vi "Main.vi"() -> ()   [LabVIEW 2014]
uses:
  <vilib>/regexp/Match Regular Expression.xnode
panel:
  out "Disticts":dbl
  in  "Find # Distincts":bool
  out "Symbol":string
  in  "Find Symbol":bool
  in  "Clear":bool
  in  "Stop Button":bool
  in  "Validate":bool
  out "Valid?":bool
  in  "Element symbol":string
  in  "Element Name":string
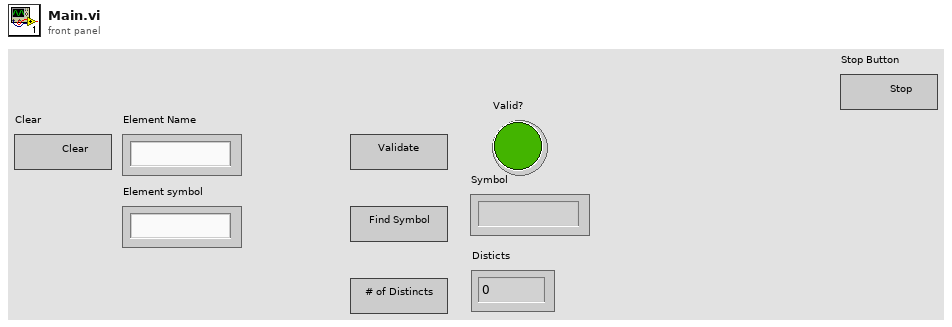
[diagram p1: front panel]
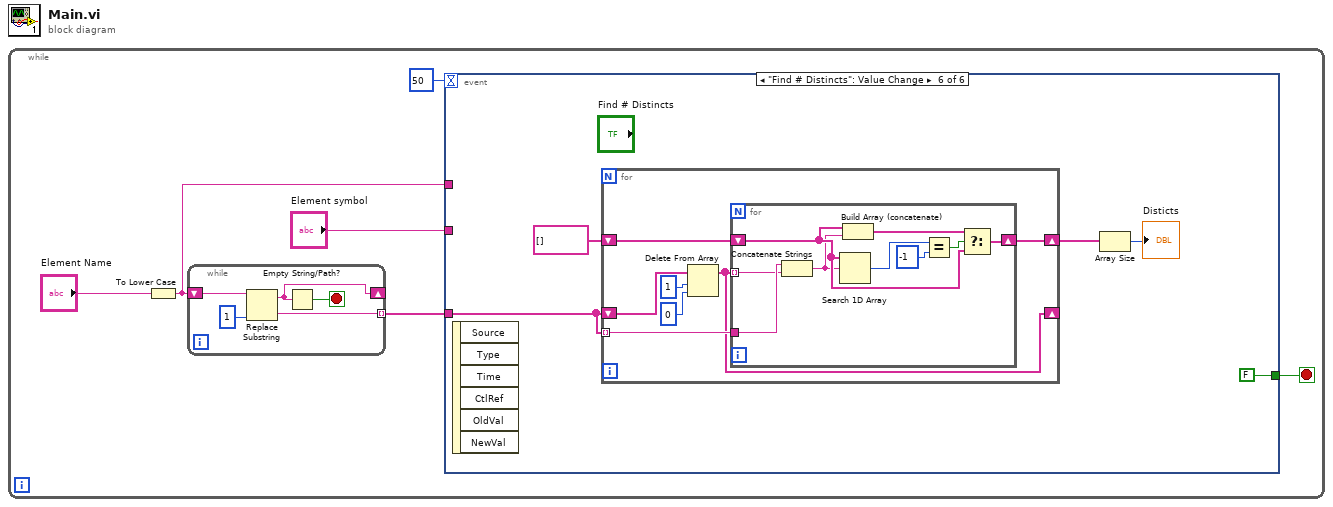
[diagram p0: block diagram]
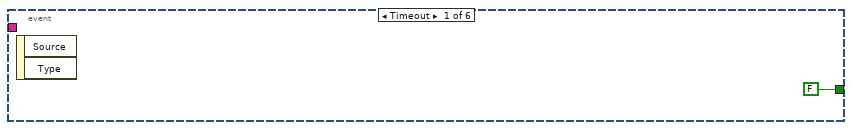
[diagram p2: hidden frame]
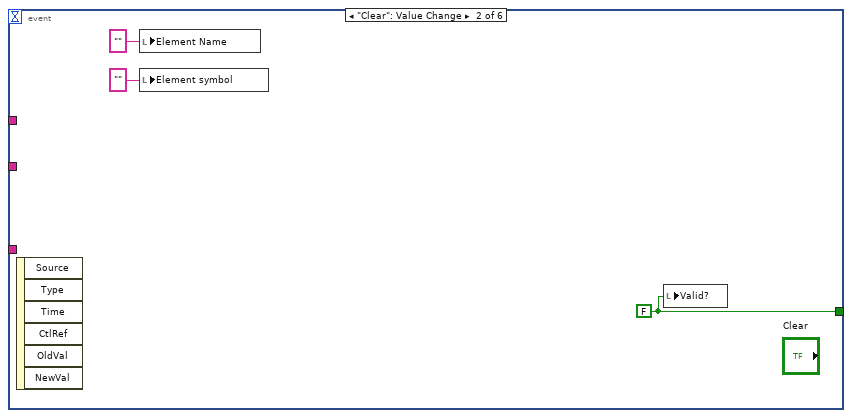
[diagram p3: hidden frame]
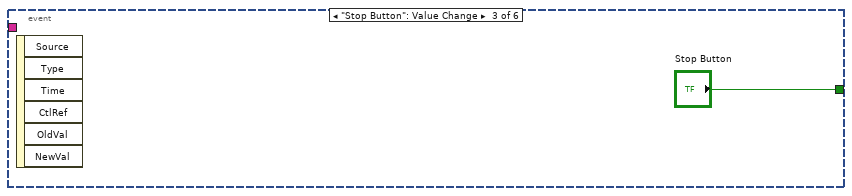
[diagram p4: hidden frame]
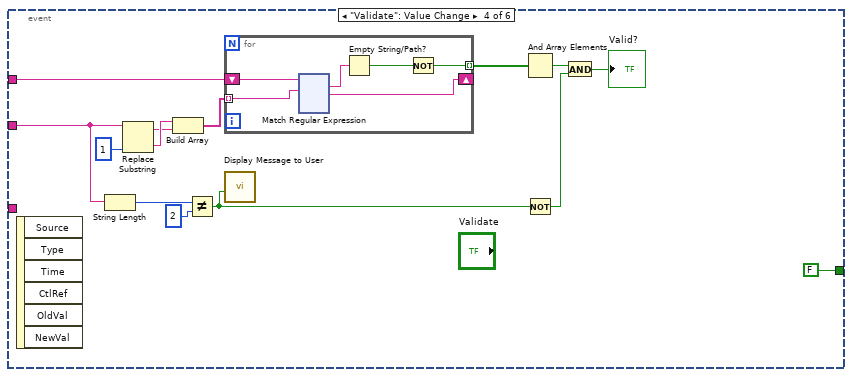
[diagram p5: hidden frame]
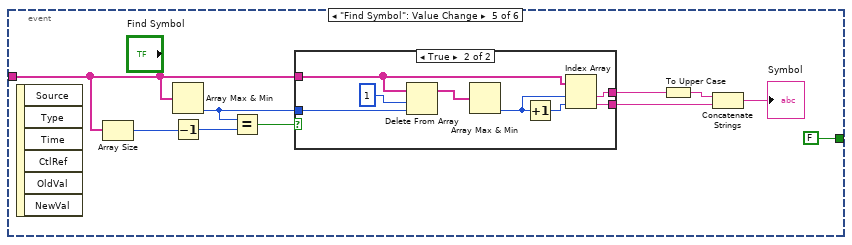
[diagram p6: hidden frame]
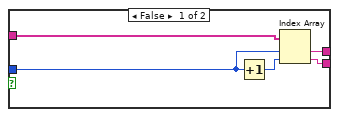
[diagram p7: hidden frame]
diagram:
  n1 = while {
    stop <- w6 stop-if-true
    n2 = To Lower Case(string="Element Name") -> (all lower case string=w2:string)
    n3 = while {
      shift-right: [w8] -> _
      shift-left: w2 -> [w11]
      tunnel: [w9] -> w1 mode=indexing
      stop <- w7 stop-if-true
      n4 = Replace Substring(2:1 ("length (len. of substring)"), 5:w11) -> (0:w9:string, 1:w8:string)  [unwired: 2 in]
      n5 = Empty String/Path?(string/path=w8) -> (empty?=w7:bool)
    }
    n6 = event shown="[5] \"Find # Distincts\": Value Change" {
      selector: _ -> [_ _ _ _ _ _]
      dyn-events: _ -> [_ _ _ _ _ _]
      timeout: 50 -> [_ _ _ _ _ _]
      tunnel: [FALSE w15 "Stop Button" FALSE ("Stop Button") FALSE ("Stop Button") FALSE ("Stop Button")] -> w6
      tunnel: w2 -> [_ _ _ w18 _ _]
      tunnel: "Element symbol" -> [_ _ _ w17 _ _]
      tunnel: w1 -> [_ _ _ _ w151 w177]
      event Timeout {
        n7 = event-data() -> ()  [unwired: 1 in, 2 out]
      }
      event "Clear": Value Change {
        w15 = FALSE
        n8 = event-data() -> ()  [unwired: 1 in, 6 out]
        n9 = local write "Element Name"("" ("Element Name")) -> ()
        n10 = local write "Element symbol"("" ("Element symbol")) -> ()
        n11 = local write "Valid?"(w15) -> ()
      }
      event "Stop Button": Value Change {
        n12 = event-data() -> ()  [unwired: 1 in, 6 out]
      }
      event "Validate": Value Change {
        n13 = event-data() -> ()  [unwired: 1 in, 6 out]
        n14 = String Length(string=w17) -> (length=w24:i32)
        n15 = Replace Substring(2:1 ("length (len. of substring)"), 5:w17) -> (0:w29:string, 1:w28:string)  [unwired: 2 in]
        n16 = Build Array(w29, w28) -> (w27:string[])
        n17 = Not Equal?(x=w24, y=2) -> (x != y?=w22:bool)
        n18 = for {
          tunnel: w27 -> [w34] mode=indexing
          shift-right: [w35] -> _
          shift-left: w18 -> [w36]
          tunnel: [w31] -> w26 mode=indexing
          n19 = xnode "Match Regular Expression"("input string"=w36, "regular expression"=w34) -> ("whole match"=w33:string, "after match"=w35:string)  [unwired: 4 in, 3 out]
          n20 = Empty String/Path?(string/path=w33) -> (empty?=w32:bool)
          n21 = Not(x=w32) -> (.not. x?=w31:bool)
        }
        n22 = call "Display Message to User"("Enable"=w22) -> ()  [unwired: 9 in, 2 out]
        n23 = And Array Elements(Boolean array=w26) -> (logical AND=w21:bool)
        n24 = Not(x=w22) -> (.not. x?=w20:bool)
        n25 = And(x=w21, y=w20) -> (x .and. y?=→"Valid?":bool)
      }
      event "Find Symbol": Value Change {
        n26 = event-data() -> ()  [unwired: 1 in, 6 out]
        n27 = Array Size(array=w151) -> (size(s)=w159:i32)
        n28 = Array Max & Min(array=w151) -> (min index (indices)=w157:i32)  [unwired: 3 out]
        n29 = Decrement(x=w159) -> (x-1=w158:i32)
        n30 = Equal?(x=w157, y=w158) -> (x = y?=w156:bool)
        n31 = case shown="True" w156 {
          tunnel: w151 -> [w161 w170]
          tunnel: w157 -> [w164 w173]
          tunnel: [w163 w167] -> w153
          tunnel: [w162 w166] -> w155
          frame False {
            n32 = Increment(x=w164) -> (x+1=w165:i32)
            n33 = Index Array(array=w161, index #1=w164, index #2=w165) -> (element #1=w163:string, element #2=w162:string)
          }
          frame True {
            n34 = Delete From Array(array=w170, length=1, index=w173) -> (array with subset deleted=w171:string[])  [unwired: 1 out]
            n35 = Array Max & Min(array=w171) -> (min index (indices)=w169:i32)  [unwired: 3 out]
            n36 = Increment(x=w169) -> (x+1=w168:i32)
            n37 = Index Array(array=w170, index #1=w169, index #2=w168) -> (element #1=w167:string, element #2=w166:string)
          }
        }
        n38 = To Upper Case(1:w153) -> (0:w152:string)
        n39 = Concatenate Strings(w152, w155) -> (→"Symbol":string)
      }
      event "Find # Distincts": Value Change {
        n40 = event-data() -> ()  [unwired: 1 in, 6 out]
        n41 = for {
          tunnel: w177 -> [w182] mode=indexing
          shift-right: [w181] -> _
          shift-left: w177 -> [w185]
          shift-right: [w179] -> w175
          shift-left: string[] [] -> [w180]
          n42 = Delete From Array(array=w185, length=1, index=0) -> (array with subset deleted=w181:string[])  [unwired: 1 out]
          n43 = for {
            tunnel: w181 -> [w193] mode=indexing
            tunnel: w182 -> [w194]
            shift-right: [w189] -> w179
            shift-left: w180 -> [w192]
            n44 = Concatenate Strings(w194, w193) -> (w191:string)
            n45 = Search 1D Array(1D array=w192, element=w191) -> (index of element=w188:i32)  [unwired: 1 in]
            n46 = Build Array (concatenate)(w192, w191) -> (w190:string[])
            n47 = Equal?(x=w188, y=-1) -> (x = y?=w186:bool)
            n48 = Select(t=w190, s=w186, f=w192) -> (s? t:f=w189:string[])
          }
        }
        n49 = Array Size(array=w175) -> (size(s)=→"Disticts":i32)
      }
    }
  }
